vi "cRIO FPGA Main.vi"() -> ()   [LabVIEW 2018]
uses:
  <vilib>/LabVIEW Targets/FPGA/cRIO/shared/nicrio_ModuleControls/nicrio_cRIO-9234_DataRatesRing2.ctl
  <vilib>/LabVIEW Targets/FPGA/cRIO/shared/nicrio_ModuleControls/nicrio_cRIO-9234_ConfigModeRing.ctl
  <vilib>/rvi/Emulation/niFpgaGetClockAttributes.vi
  <vilib>/rvi/Emulation/niFpgaSctlEmulationGetInTimedLoop.vi
  <vilib>/rvi/Emulation/niFpgaEmulationReportErrorSimple.vi
  <vilib>/rvi/eio/common/nirviEmuTemplateMethod_errors.vi
  <vilib>/rvi/Emulation/niFpgaCriticalErrorInLSC.vi
  <vilib>/rvi/eio/common/nirviEmuTemplatePropertySet_errors.vi
  <vilib>/rvi/interface/RandomDataEmulation/niFpgaRandomDataHandleErrors.vi
  <vilib>/eio/EIONode/EIONode.xnode
  <vilib>/eio/EIOPropertyNode/EIOPropertyNode.xnode
  <vilib>/rvi/DataTransferAndStorage/Container/XNode/niFpgaContainer.xnode
  <vilib>/rvi/interface/RandomDataEmulation/nirviRandomDataFpgaReadWriteTemplate.vi
  <vilib>/rvi/eio/common/nirviEmuTemplatePropertyGet_errors.vi
  <vilib>/rvi/eio/common/nirviEmuTemplatePropertyGet_noerrors.vi
  <vilib>/rvi/eio/common/nirviEmuTemplatePropertySet_noerrors.vi
panel:
  out "Data FIFO Full":bool
  out "00-03-9402 (RPM)":sgl[](array[numeric])
  in  "Accelerometer Configs":T1[](array[typedef])=[2, 2, 2, 2] items=["AC Coupled", "DC Coupled", "IEPE AC Coupled"]
  in  "Data Rate":T2=1 items=["51.200 kS/s (NI 9234)"=1, "25.600 kS/s (NI 9234)"=2, "17.067 kS/s (NI 9234)"=3, "12.800 kS/s (NI 9234)"=4, "10.240 kS/s (NI 9234)"=5, "8.533 kS/s (NI 9234)"=6, "7.314 kS/s (NI 9234)"=7, "6.400 kS/s (NI 9234)"=8, "5.689 kS/s (NI 9234)"=9, "5.120 kS/s (NI 9234)"=10, "4.654 kS/s (NI 9234)"=11, "4.267 kS/s (NI 9234)"=12, "3.938 kS/s (NI 9234)"=13, "3.657 kS/s (NI 9234)"=14, "3.413 kS/s (NI 9234)"=15, "3.200 kS/s (NI 9234)"=16, "3.012 kS/s (NI 9234)"=17, "2.845 kS/s (NI 9234)"=18, "2.695 kS/s (NI 9234)"=19, "2.560 kS/s (NI 9234)"=20, "2.438 kS/s (NI 9234)"=21, "2.328 kS/s (NI 9234)"=22, "2.226 kS/s (NI 9234)"=23, "2.133 kS/s (NI 9234)"=24, "2.048 kS/s (NI 9234)"=25, "1.969 kS/s (NI 9234)"=26, "1.896 kS/s (NI 9234)"=27, "1.829 kS/s (NI 9234)"=28, "1.765 kS/s (NI 9234)"=29, "1.707 kS/s (NI 9234)"=30, "1.652 kS/s (NI 9234)"=31]
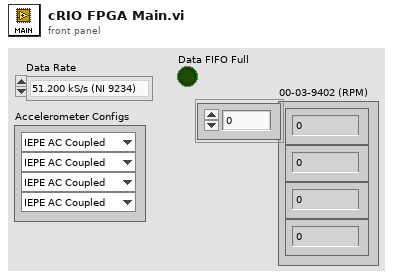
[diagram p1: front panel]
types:
  T1 = typedef "nicrio_cRIO-9234_ConfigModeRing.ctl" = u8
  T2 = typedef "nicrio_cRIO-9234_DataRatesRing2.ctl" = u8
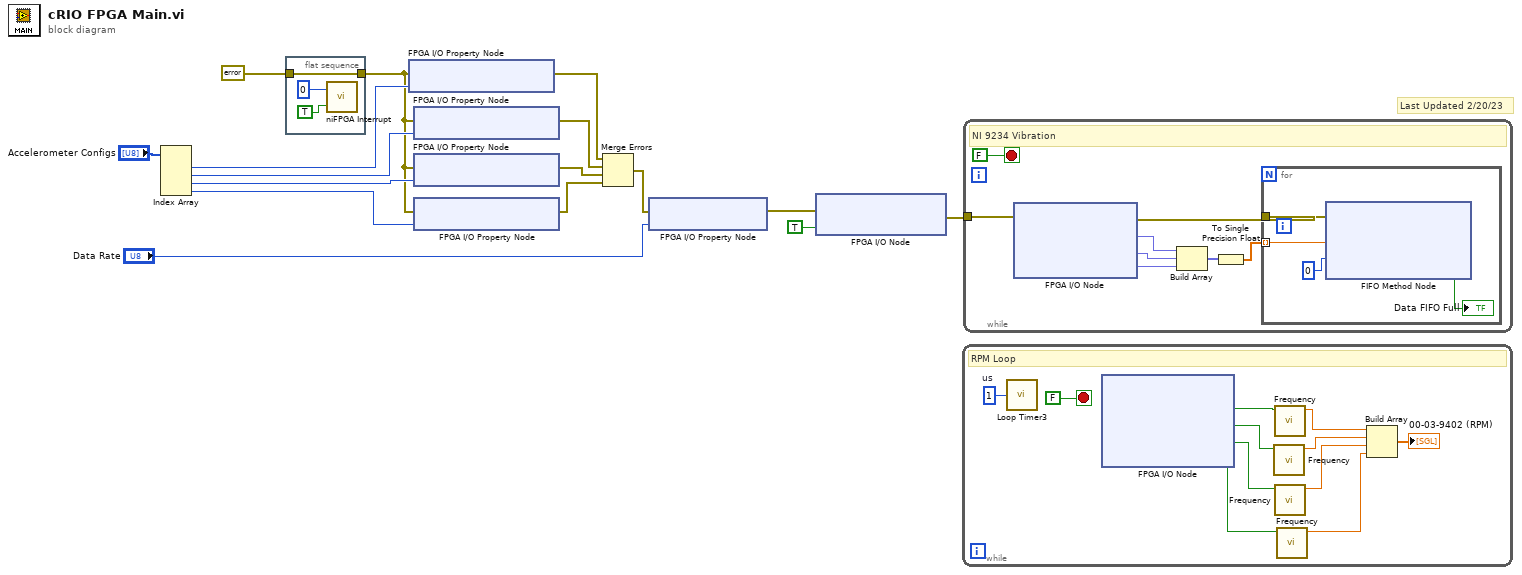
[diagram p0: block diagram]
diagram:
  # "Last Updated 2/20/23"
  n1 = Index Array(array="Accelerometer Configs") -> (element #1=w13:T1, element #2=w12:T1, element #3=w11:T1, element #4=w10:T1)  [unwired: 4 in]
  n2 = flat-sequence {
    tunnel: errorcluster {"status"=FALSE, "code"=0, "source"=""} ("error out") -> [w17]
    tunnel: [w17] -> w3
    frame #0 {
      n3 = call <vilib>:"niFPGA Interrupt.vi"("Wait Until Cleared (F)"=TRUE ("Wait Until Cleared"), "IRQ Number (0)"=u8 0 ("IRQ Bit (0-31)")) -> ()  [unwired: 1 in]
    }
  }
  n4 = xnode "FPGA I/O Property Node"("error in"=w3, "Input Configuration"=w13) -> ("error out"=w6:errorcluster)  [unwired: 1 in, 1 out]
  n5 = xnode "FPGA I/O Property Node"("error in"=w3, "Input Configuration"=w12) -> ("error out"=w7:errorcluster)  [unwired: 1 in, 1 out]
  n6 = xnode "FPGA I/O Property Node"("error in"=w3, "Input Configuration"=w11) -> ("error out"=w8:errorcluster)  [unwired: 1 in, 1 out]
  n7 = xnode "FPGA I/O Property Node"("error in"=w3, "Input Configuration"=w10) -> ("error out"=w9:errorcluster)  [unwired: 1 in, 1 out]
  n8 = Merge Errors(w6, w7, w8, w9) -> (w5:errorcluster)
  n9 = xnode "FPGA I/O Property Node"("error in"=w5, "Data Rate"="Data Rate") -> ("error out"=w2:errorcluster)  [unwired: 1 in, 1 out]
  n10 = xnode "FPGA I/O Node"("error in"=w2, "00-02-9234/Start"=TRUE) -> ("error out"=w1:errorcluster)  [unwired: 1 in, 1 out]
  n11 = while {
    stop <- FALSE stop-if-true
    w30 = u32 1  # us
    # "RPM Loop"
    n12 = call "Loop Timer3"("Count(uSec)"=w30) -> ()  [unwired: 1 out]
    n13 = xnode "FPGA I/O Node"() -> ("00-03-9402/DIO0"=w28:bool, "00-03-9402/DIO1"=w27:bool, "00-03-9402/DIO2"=w26:bool, "00-03-9402/DIO3"=w25:bool)  [unwired: 5 in, 5 out]
    n14 = call "Frequency.vi"("New Value"=w27) -> ("RPM"=w23:sgl)  [unwired: 10 in]
    n15 = call "Frequency.vi"("New Value"=w28) -> ("RPM"=w24:sgl)  [unwired: 10 in]
    n16 = call "Frequency.vi"("New Value"=w26) -> ("RPM"=w22:sgl)  [unwired: 10 in]
    n17 = call "Frequency.vi"("New Value"=w25) -> ("RPM"=w21:sgl)  [unwired: 10 in]
    n18 = Build Array(w24, w23, w22, w21) -> (→"00-03-9402 (RPM)":sgl[])
  }
  n19 = while {
    tunnel: w1 -> [w32]
    stop <- FALSE stop-if-true
    # "NI 9234 Vibration"
    n20 = xnode "FPGA I/O Node"("error in"=w32) -> ("error out"=w31:errorcluster, "00-02-9234/AI0"=w33:fxp<+/-,24,4>, "00-02-9234/AI1"=w34:fxp<+/-,24,4>, "00-02-9234/AI2"=w35:fxp<+/-,24,4>)  [unwired: 3 in, 3 out]
    n21 = Build Array(w33, w34, w35) -> (w37:fxp<+/-,24,4>[])
    n22 = To Single Precision Float(number=w37) -> (single precision float=w36:sgl[])
    n23 = for {
      tunnel: w36 -> [w40] mode=indexing
      tunnel: w31 -> [w41]
      n24 = xnode ("FIFO Method Node")("Element"=w40, "Timeout"=0, "error in (no error)"=w41) -> ("Timed Out?"=→"Data FIFO Full":bool)  [unwired: 1 in, 2 out]
    }
  }
